vi "class discovery singleton.vi"(6 "Folders to Exclude":string[](array[string]), 8 "error in":errorcluster, 9 "Plugin Search Paths":path[](array[path]), 10 "Class Name":string, 11 "method":T1) -> (0 "error out":errorcluster, 1 "class path":path, 2 "LabVIEW Object":refnum<class>, 4 "discovered classes":path[](array[path]))   [LabVIEW 2013, in "class discovery singleton.lvlib"]
doc: "A functional global variable which provides name-based lookup of classes. When a search path is added, the FGV will locate all classes on disk and use the *filename* to cache them in memory. That is, the class c:\\classes\\foo.lvclass is stored as foo, not as FrameworkClasses.lvlib::Foo.lvclass. The assumption is that anything already in memory can be loaded by other means. When a load is requested, the FGV will first use the name as an input to get lvclass default value by name (which does expect FrameworkClasses.lvlib::Foo.lvclass). Then it will look for foo.lvclass in the list of found classes on disk. Then if all else fails, it will attempt to match a class in memory using a string match."
uses:
  class discovery singleton.lvlib
  class discovery singleton methods.ctl
  root configuration/TBM configuration.lvclass
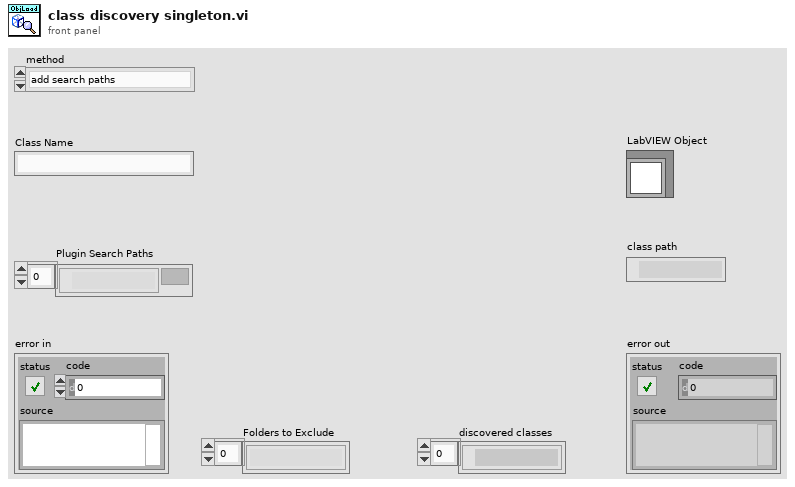
[diagram p1: front panel]
types:
  T1 = typedef "class discovery singleton.lvlib/class discovery singleton methods.ctl" = enum16{"add search paths", "load class by name", "list available classes", "get class path"}
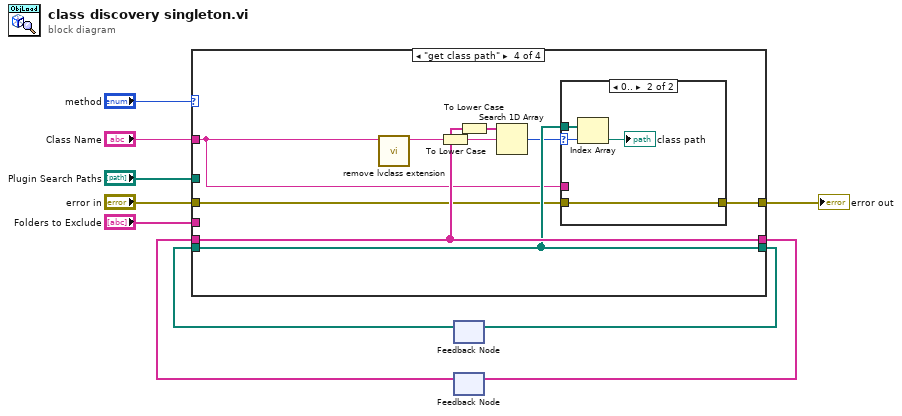
[diagram p0: block diagram]
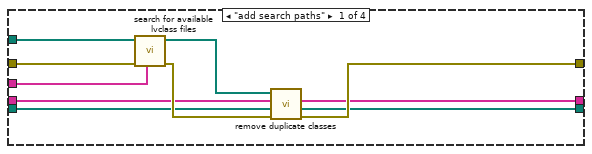
[diagram p2: hidden frame]
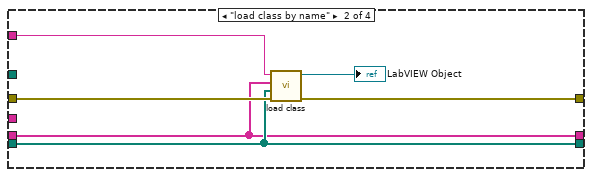
[diagram p3: hidden frame]
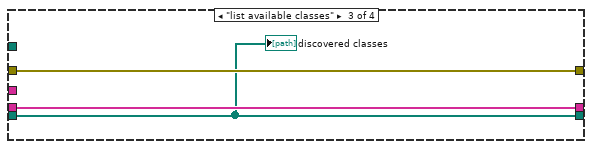
[diagram p4: hidden frame]
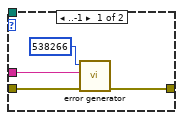
[diagram p5: hidden frame]
diagram:
  n1 = feedback #1() -> (w3:path[])  [unwired: 1 in]
  n2 = feedback #2() -> (w5:string[])  [unwired: 1 in]
  n3 = case shown="\"get class path\"" "method" {
    tunnel: "error in" -> [w20 w26 w28 w34]
    tunnel: "Plugin Search Paths" -> [w19 _ _ _]
    tunnel: [w16 w25 w28 w33] -> w7
    tunnel: w5 -> [w15 w23 w29 w38]
    tunnel: [w14 w23 w29 w38] -> w6
    tunnel: [w13 w24 w27 w36] -> w4
    tunnel: w3 -> [w12 w24 w27 w36]
    tunnel: "Class Name" -> [_ w22 _ w32]
    tunnel: "Folders to Exclude" -> [w11 _ _ _]
    frame "add search paths" {
      n4 = call "search for available lvclass files.vi"("Folders to Exclude"=w11, "error in"=w20, "Plugin Search Paths"=w19) -> ("error out"=w17:errorcluster, "discovered classes"=w18:path[])  [unwired: 7 in]
      n5 = call "remove duplicate classes.vi"("error in"=w17, "class paths in"=w12, "class names in"=w15, "discovered classes"=w18) -> ("error out"=w16:errorcluster, "class paths out"=w13:path[], "class names out"=w14:string[])  [unwired: 5 in]
    }
    frame "load class by name" {
      n6 = call "load class.vi"("error in"=w26, "available class paths"=w24, "available class names"=w23, "Class Name"=w22) -> ("error out"=w25:errorcluster, "Object Out"=→"LabVIEW Object":refnum<class>)  [unwired: 6 in]
    }
    frame "list available classes" {
      "discovered classes" <- w27
    }
    frame "get class path" {
      n7 = call "remove lvclass extension.vi"("class name in"=w32) -> ("class name out"=w31:string)  [unwired: 10 in]
      n8 = To Lower Case(string=w31) -> (all lower case string=w30:string)
      n9 = To Lower Case(string=w38) -> (all lower case string=w37:string[])
      n10 = Search 1D Array(1D array=w37, element=w30) -> (index of element=w35:i32)  [unwired: 1 in]
      n11 = case shown="0.." w35 {
        selector: w35 -> [_ w45]
        tunnel: w36 -> [_ w46]
        tunnel: w34 -> [w40 w44]
        tunnel: [w41 w44] -> w33
        tunnel: w32 -> [w39 _]
        frame ..-1 {
          n12 = call "error generator.vi"("error in"=w40, "append error message"=w39, "error code (0)"=538266) -> ("error out"=w41:errorcluster)  [unwired: 8 in]
        }
        frame 0.. {
          n13 = Index Array(array=w46, index=w45) -> (element=→"class path":path)
        }
      }
    }
  }
  "error out" <- w7
  n14 = feedback-in #1(w4) -> ()
  n15 = feedback-in #2(w6) -> ()
